vi "OPC and SRQ test.vi"() -> ()   [LabVIEW 2018]
uses:
  <vilib>/Instr/_visa.llb/Select Event Type.ctl
panel:
  in  "VISA GPIB Resource":refnum<visa-resource-name>="GPIB0::3::INSTR"
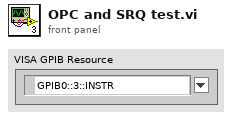
[diagram p1: front panel]
types:
  T1 = typedef "Select Event Type.ctl" = u32
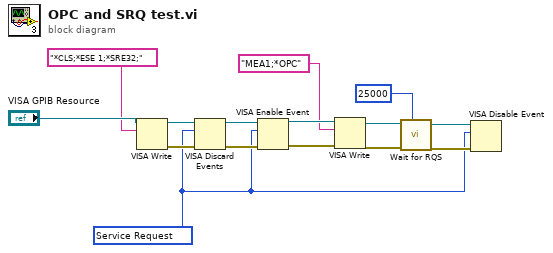
[diagram p0: block diagram]
diagram:
  w1 = T1 1073684491 items=["Service Request"=1073684491, "Trigger"=3221168138, "Clear"=1073684493, "VXI Signal"=1073684512, "VXI/VME Interrupt"=3221168161, "VXI/VME Sysfail"=1073684509, "VXI/VME Sysreset"=1073684510, "GPIB CIC"=1073684498, "GPIB Talk"=1073684499, "GPIB Listen"=1073684500, "PXI Interrupt"=1073684514, "Serial Break"=1073684515, "Serial TermChar"=1073684516, "Serial CTS"=1073684521, "Serial DSR"=1073684522, "Serial DCD"=1073684524, "Serial RI"=1073684526, "Serial Character"=1073684533, "USB Interrupt"=1073684535, "All Enabled"=1073709055] ("Event Type")
  n1 = VISA Write(VISA resource name="VISA GPIB Resource", write buffer="*CLS;*ESE 1;*SRE32;") -> (VISA resource name out=w12:refnum<visa-resource-name>, error out=w13:errorcluster)  [unwired: 1 in, 1 out]
  n2 = VISA Discard Events(8:w13, 10:w1, 11:w12) -> (0:w10:errorcluster, 3:w11:refnum<visa-resource-name>)  [unwired: 1 in]
  n3 = VISA Enable Event(8:w10, 10:w1, 11:w11) -> (0:w8:errorcluster, 3:w9:refnum<visa-resource-name>)  [unwired: 1 in]
  n4 = VISA Write(VISA resource name=w9, write buffer="MEA1;*OPC", error in (no error)=w8) -> (VISA resource name out=w6:refnum<visa-resource-name>, error out=w5:errorcluster)  [unwired: 1 out]
  n5 = call <vilib>:"Wait for RQS.vi"("timeout (25000 ms)"=u32 25000, "error in (no error)"=w5, "VISA resource name"=w6) -> ("error out"=w2:errorcluster, "VISA resource name out"=w3:refnum<visa-resource-name>)  [unwired: 6 in, 1 out]
  n6 = VISA Disable Event(8:w2, 10:w1, 11:w3) -> ()  [unwired: 1 in, 2 out]
